vi "ROI entry-Offset mode colour.vi"(8 "error in (no error)":errorcluster) -> (0 "error out":errorcluster)   [LabVIEW 2017]
uses:
  Globals/gl_ROI Entry UI globals.vi
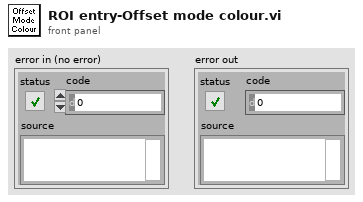
[diagram p1: front panel]
types:
  T1 = typedef "ROI entry screen ctrl refs cluster.ctl" = cluster{"Done button":refnum<vi>, "Imaging button":refnum<vi>, "Acquisition button":refnum<vi>, "POI dwell time (us)":refnum<vi>, "Scan dwell time per pixel (us)":refnum<vi>, "# of planes":refnum<vi>, "Zoom Ctrl":refnum<vi>, "Equal size":refnum<vi>, "Channel":refnum<vi>, "Image Display":refnum<vi>, "Z-Plane Selector":refnum<vi>, "Number of lines left":refnum<vi>, "Z-stack folder path":refnum<vi>, "POI Density":refnum<vi>, "Arb Plane Entry":refnum<vi>, "Whole plane":refnum<vi>, "Clear Last":refnum<vi>, "Clear All":refnum<vi>, "Trial Length (sec)":refnum<vi>, "Palette Type":refnum<vi>, "Intensity slider":refnum<vi>, "# POI":refnum<vi>, "Max Z Proj":refnum<vi>, "Zplane ind":refnum<vi>, "Wavelength (nm)":refnum<vi>, "Number of Trials":refnum<vi>, "Funct stim.trig.enable":refnum<vi>, "Funct stim.trig.delay (s)":refnum<vi>, "Line Mode":refnum<vi>, "Step size (µm)":refnum<vi>, "ROI move mode":refnum<vi>, "Cool-down time (s)":refnum<vi>, "Enable cool-down time":refnum<vi>, "Motor Z ind. (um)":refnum<vi>, "AOL Z ind. (um)":refnum<vi>, "Load Reference Image":refnum<vi>}
  T2 = typedef "ROI move mode.ctl" = enum16{"ROI on ALL planes", "ROI on current plane"}
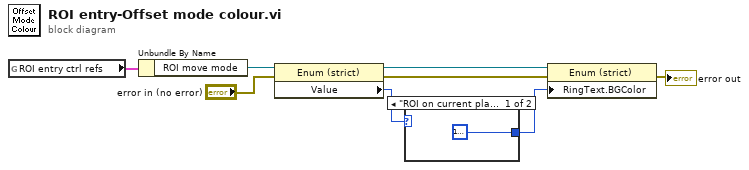
[diagram p0: block diagram]
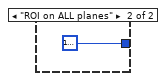
[diagram p2: hidden frame]
diagram:
  n1 = global read "gl_ROI Entry UI globals.vi" "ROI entry ctrl refs"() -> (w4:T1)
  n2 = Unbundle By Name(w4) -> ("ROI move mode"=w5:refnum<vi>)
  n3 = property on="Property Node" class="Enum (strict)"(reference=w5, error in="error in (no error)") -> (reference out=w7:refnum<vi>, error out=w1:errorcluster, "Value"=w6:T2)
  n4 = case shown="\"ROI on current plane\"" w6 {
    tunnel: [u32 16777216 u32 16777216] -> w8
    frame "ROI on current plane" {
    }
    frame "ROI on ALL planes" {
    }
  }
  n5 = property on="Property Node" class="Enum (strict)"(reference=w7, error in=w1, "RingText.BGColor"=w8) -> (error out=→"error out":errorcluster)  [unwired: 1 out]
